vi "add.vi"() -> ()   [LabVIEW 2025]
panel:
  in  "d":dbl
  out "c":dbl
  in  "b":dbl
  in  "a":dbl
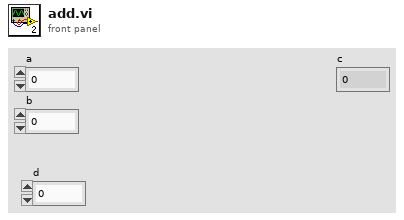
[diagram p1: front panel]
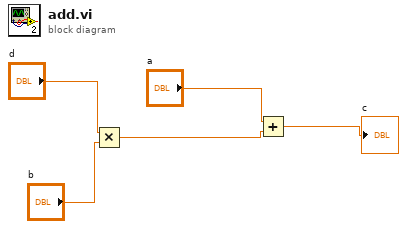
[diagram p0: block diagram]
diagram:
  n1 = Multiply(x="d", y="b") -> (x*y=w1:dbl)
  n2 = Add(x="a", y=w1) -> (x+y=→"c":dbl)
